vi "Create Server.vi"(8 "error in":errorcluster) -> (0 "error out":errorcluster, 3 "gRPCid out":T1)   [LabVIEW 2020, in "grpc-lvsupport-release.lvlib"]
uses:
  gRPC Data Server Engine Windows.llb/grpc-lvsupport-release.lvlib
  gRPC Data Server Engine Windows.llb/grpcId.ctl
  gRPC Data Server Engine Windows.llb/Error Cluster From Error Code.vi
  gRPC Data Server Engine Windows.llb/Simple Error Handler.vi
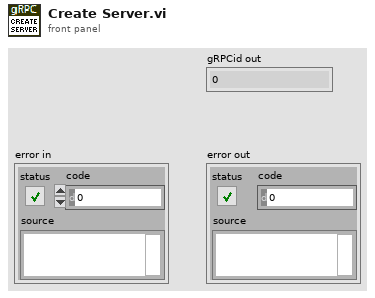
[diagram p1: front panel]
types:
  T1 = typedef "grpc-lvsupport-release.lvlib/grpcId.ctl" = u64
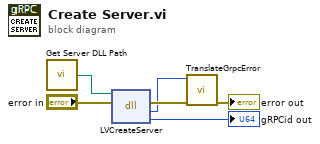
[diagram p0: block diagram]
diagram:
  n1 = call "Get Server DLL Path.vi"() -> ("Server dll path"=w3:path)
  n2 = dll-call lib="C:/Users/XEnderMD/Desktop/LV gRPC/labview source/gRPC interface/dlls/labview_grpc_server.dll" fn="LVCreateServer"(path in=w3, error in="error in") -> (error out=w5:errorcluster, "return type"=w1:i32, "gRPCid out"=→"gRPCid out":T1)  [unwired: 2 in, 1 out]
  n3 = call "TranslateGrpcError.vi"("error in"=w5, "Error Code"=w1) -> ("error out"=→"error out":errorcluster)  [unwired: 9 in]
